vi "Deinterleave.vi"(0 "device session in":refnum<class "Device Session.lvclass">, 5 "target data in":i16[][](array[numeric]), 7 "source data":refnum<data-value>, 11 "error in":errorcluster) -> (4 "device session out":refnum<class "Device Session.lvclass">, 6 "target data out":i16[][](array[numeric]), 15 "error out":errorcluster)   [LabVIEW 2015, in "Device Session.lvclass"]
doc: "Takes in a two-dimensional array and a fetched sample data value reference and deinterleaves the fetched samples into the array.\n\n<B>Input Parameters</B>\n\n<B>device session in</B> is a reference to the session containing sessions to all instrument design libraries used in this sample project. This parameter is obtained from the 'Open Session' VI.\n\n<B>target data in</B> specifies the target array to receive the deinterleaved data. This array should be created in the 'Create Deinterleave Sample Buffer'.\n\n<B>source data</B> specifies the data value reference of fetched samples returned from the 'Fetch Data DVR' VI.\n\n<B>error in</B> describes error conditions that occur before this node runs. This input provides standard 'error in' functionality.\n\n<B>Output Parameters</B>\n\n<B>device session out</B> passes a reference to the session to the next VI.\n\n<B>target data out</B> returns the two-dimensional array with deinterleaved sample data.\n\n<B>error out</B> contains error information. This output provides standard 'error out' functionality."
uses:
  Device Session.lvclass
  Device Session.lvclass/Device Session.ctl
  <instrlib>/_niInstr/Data Manipulation/v1/Host/Private/Deinterleave I161D to I162D.vi
  <instrlib>/_niInstr/Data Manipulation/v1/Host/Private/Map C Error to DataManip Error.vi
  <instrlib>/_niInstr/Data Manipulation/v1/Host/Private/Data Manipulation Error Handler.vi
  <instrlib>/_niInstr/Data Manipulation/v1/Host/niInstr Data Manipulation v1 Host.lvlib
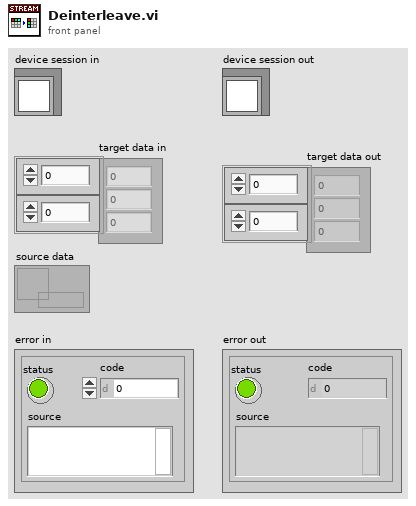
[diagram p1: front panel]
types:
  T1 = typedef "Device Session.lvclass/Device Session Object.ctl" = cluster{"ni5171R FPGA Reference":T2, "niHSAI config":refnum<class "niHSAI Config v1 Host.lvclass">, "configured scaling coefficients":cluster{"gain":dbl, "offset":dbl}[], "number of channels to stream":u8, "selected acq channels":bool[], "number of channels":u32, "actual channel configuration":T3[], "configured channels":bool[], "sample clock rate (Hz)":dbl}
  T2 = typedef "Device Session.lvclass/FPGA Refnum.ctl" = refnum<k20>
  T3 = typedef "niHSAI Types v1 Host.lvlib/Channel Configuration.ctl" = cluster{"channel":u32, "coupling":T4, "impedance":T5, "bandwidth":T6, "vertical range":dbl, "vertical offset":dbl}
  T4 = typedef "niHSAI Types v1 Host.lvlib/Coupling.ctl" = enum8{"Default", "DC", "AC"}
  T5 = typedef "niHSAI Types v1 Host.lvlib/Impedance.ctl" = enum8{"Default", "1 mega ohm", "50 ohm"}
  T6 = typedef "niHSAI Types v1 Host.lvlib/Bandwidth.ctl" = enum8{"Default", "Full Bandwidth", "Anti-alias Filter"}
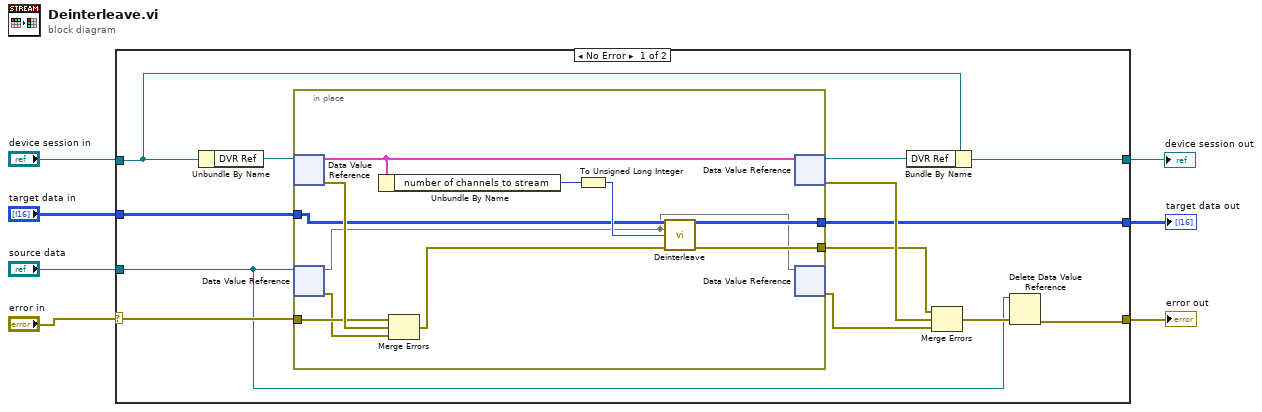
[diagram p0: block diagram]
diagram:
  n1 = case shown="No Error" "error in" {
    selector: "error in" -> [w20 w34]
    tunnel: "device session in" -> [w17 w33]
    tunnel: [w16 w33] -> w6
    tunnel: [w9 w34] -> w1
    tunnel: "source data" -> [w8 _]
    tunnel: "target data in" -> [w14 w32]
    tunnel: [w13 w32] -> w2
    frame No Error {
      n2 = Unbundle By Name(w17) -> ("DVR Ref"=w19:refnum<data-value>)
      n3 = in-place {
        in-place-border: w20 -> [w29]
        in-place-border: w14 -> [w25]
        in-place-border: [w23] -> w13
        in-place-border: [w22] -> w12
        n4 = in-place-dvr #1(w19) -> (w31:T1, w30:errorcluster)
        n5 = in-place-dvr #2(w8) -> (w21:i16[], w24:errorcluster)
        n6 = Unbundle By Name(w31) -> ("number of channels to stream"=w28:u8)
        n7 = Merge Errors(w29, w30, w24) -> (w26:errorcluster)
        n8 = To Unsigned Long Integer(number=w28) -> (unsigned 32bit integer=w27:u32)
        n9 = call-poly <instrlib>:"Deinterleave.vi"("data in"=w25, "new data"=w21, "deinterleave factor"=w27, "error in"=w26) -> ("data out"=w23:i16[][], "error out"=w22:errorcluster)  [unwired: 8 in, 2 out]
        n10 = in-place-dvr #1(w31) -> (w18:refnum<data-value>, w15:errorcluster)
        n11 = in-place-dvr #2(w21) -> (w11:errorcluster)  [unwired: 1 out]
      }
      n12 = Bundle By Name(cluster=w17, "DVR Ref"=w18) -> (w16:refnum<class "Device Session.lvclass">)
      n13 = Merge Errors(w12, w15, w11) -> (w10:errorcluster)
      n14 = Delete Data Value Reference(data value reference=w8, error in=w10) -> (error out=w9:errorcluster)  [unwired: 1 out]
    }
    frame Error {
    }
  }
  "target data out" <- w2
  "error out" <- w1
  "device session out" <- w6
